vi "PH_gentec_P-Link.Action get and set current Settings for the first Time.vi"(0 "i ref in":refnum<vi>, 5 "error in":errorcluster) -> (14 "i ref out":refnum<vi>, 19 "error out":errorcluster)   [LabVIEW 2014, in "PH_gentec_P-Link.lvlib"]
doc: "This VI gets and sets all current settings for the first time."
uses:
  PH_gentec_P-Link.lvlib
  PH_Basics/PH_Powermeter_BaseClass/PH_Powermeter_BaseClass.State.ctl
  PH_Basics/PH_Powermeter_BaseClass/PH_gentec_BaseClass.Head Settings.ctl
  PH_Basics/PH_Powermeter_BaseClass/PH_Powermeter_BaseClass.lvlib
  instr.lib/Gentec-P-Link/gentec-P-Link - Driver.lvlib
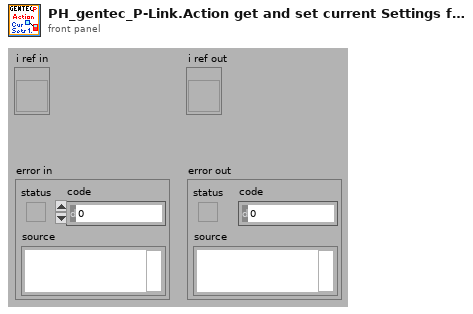
[diagram p1: front panel]
types:
  T1 = typedef "PH_Powermeter_BaseClass.lvlib/PH_gentec_BaseClass.Head Settings.ctl" = cluster{"Trigger Level":dbl, "Wavelength":u32, "Range":u32}
  T2 = typedef "PH_Powermeter_BaseClass.lvlib/PH_Powermeter_BaseClass.State.ctl" = enum32{"off", "operating", "opened", "checked", "connected", "Sets to change", "running"}
  T3 = typedef "PH_Powermeter_BaseClass.lvlib/PH_Powermeter_BaseClass.i attribute.ctl" = cluster{"GUI References":T4, "Connection":T5, "Head Attributes":T6, "VISA resource":refnum<visa-resource-name>, "Energy":T7, "Service ID Energy":i32, "Wanted Settings":T1, "Current Settings":T1}
  T4 = typedef "PH_Powermeter_BaseClass.lvlib/PH_Powermeter_BaseClass.GUI Refs.ctl" = cluster{"Head Attributes":refnum<vi>, "Energy":refnum<vi>, "Connection":refnum<vi>, "VISA Resource":refnum<vi>, "Scaling Factor":refnum<vi>, "Range":refnum<vi>, "Wavelength":refnum<vi>, "Trigger Level":refnum<vi>, "Wanted Settings":refnum<vi>, "Current Settings":refnum<vi>}
  T5 = typedef "PH_Powermeter_BaseClass.lvlib/PH_Powermeter_BaseClass.Connection.ctl" = cluster{"failed checks":i8, "Timeout":bool, "Data read":string, "Failure":bool, "Error":bool, "State":T2}
  T6 = typedef "PH_Powermeter_BaseClass.lvlib/PH_Powermeter_BaseClass.Head Attributes.ctl" = cluster{"Instrument Type":string, "Head Version":string, "Head Name":string, "Serial Number":string, "Firmware":string, "Sensor Type":string, "MinimumRange":u32, "Maximum Range":u32, "Min Wavelength":i32, "Max Wavelength":i32}
  T7 = typedef "PH_Powermeter_BaseClass.lvlib/PH_Powermeter_BaseClass.Energy.ctl" = cluster{"current Value":dbl, "unscaled":dbl, "Scaling Factor":dbl}
  T8 = typedef "PH_gentec_P-Link.lvlib/PH_gentec_P-Link.i attribute.ctl" = cluster{"GUI References":cluster{"Wanted Head Settings":refnum<vi>, "Current Head Settings":refnum<vi>, "Set Auto Range":refnum<vi>, "Trigger Polarity":refnum<vi>, "Trigger Source":refnum<vi>, "Waveform Averages":refnum<vi>, "Continuous":refnum<vi>, "get one Value":refnum<vi>, "Set Zero":refnum<vi>}, "Wanted Head Settings":T9, "Current Head Settings":T9}
  T9 = typedef "PH_gentec_P-Link.lvlib/PH_gentec_P-Link.Head Settings.ctl" = cluster{"Enable Anticipation":bool, "Set Auto Range":bool, "Set Zero":i32, "Current":i32, "Start Data Flow":bool}
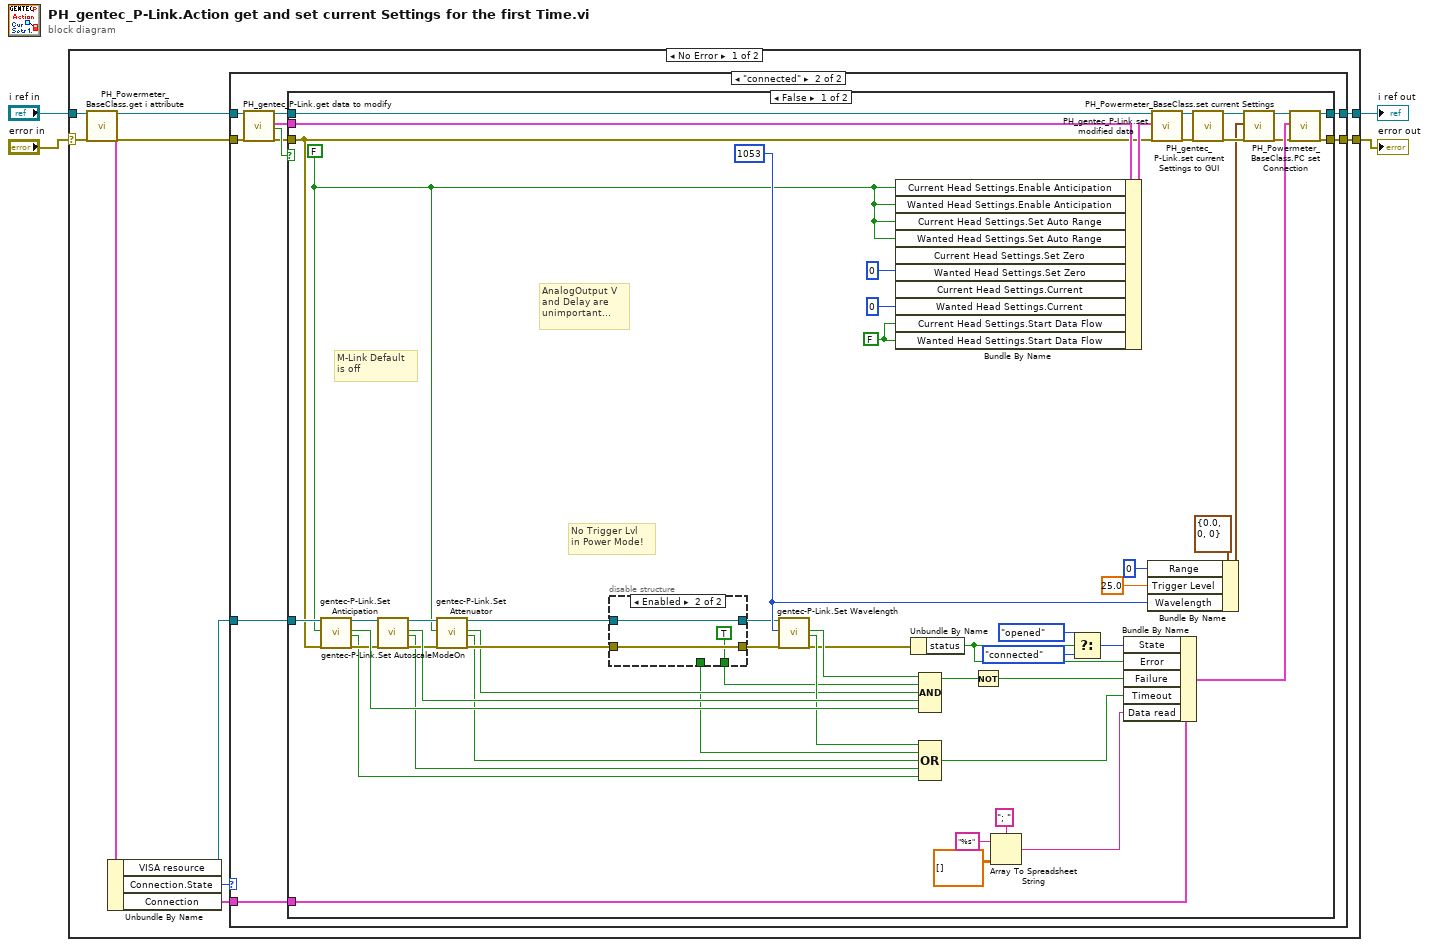
[diagram p0: block diagram]
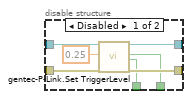
[diagram p3: hidden frame]
diagram:
  n1 = case shown="No Error" "error in" {
    selector: "error in" -> [w5 w93]
    tunnel: [w14 w93] -> w4
    tunnel: [w13 w94] -> w3
    tunnel: "i ref in" -> [w12 w94]
    frame No Error {
      n2 = call "PH_Powermeter_BaseClass.get i attribute.vi"("i ref in"=w12, "error in (no error)"=w5) -> ("i ref out"=w8:refnum<vi>, "i attribute"=w11:T3, "error out"=w7:errorcluster)  [unwired: 15 in]
      n3 = Unbundle By Name(w11) -> ("VISA resource"=w6:refnum<visa-resource-name>, "Connection.State"=w10:T2, "Connection"=w9:T5)
      n4 = case shown="\"connected\"" w10 {
        tunnel: [w15 w17] -> w14
        tunnel: [w16 w18] -> w13
        tunnel: w6 -> [_ w22]
        tunnel: w8 -> [w16 w21]
        tunnel: w7 -> [w15 w20]
        tunnel: w9 -> [_ w19]
        frame Default {
        }
        frame "connected" {
          n5 = call "PH_gentec_P-Link.get data to modify.vi"("i ref in"=w21, "error in (no error)"=w20) -> ("i ref out"=w24:refnum<vi>, "i attribute"=w25:T8, "timed out"=w26:bool, "error out"=w23:errorcluster)  [unwired: 14 in]
          n6 = case shown="False" w26 {
            tunnel: w22 -> [w61 _]
            tunnel: [w66 w92] -> w18
            tunnel: [w65 w91] -> w17
            tunnel: w23 -> [w60 w91]
            tunnel: w24 -> [w80 w92]
            tunnel: w25 -> [w77 _]
            tunnel: w19 -> [w71 _]
            frame False {
              w28 = 0 ("Current Head Settings.Current Measurement")
              w29 = FALSE ("Current Head Settings.Start Data Flow")
              w40 = u16 1053 ("Lambda")
              w27 = 0 ("Current Head Settings.Set Zero")
              w30 = FALSE ("Enable Anticipation")
              # "No Trigger Lvl\nin Power Mode!"
              # "AnalogOutput V\nand Delay are\nunimportant..."
              # "M-Link Default\nis off"
              n7 = call "gentec-P-Link.Set Anticipation.vi"("VISA resource name"=w61, "On/Off"=w30, "error in (no error)"=w60) -> ("VISA resource name"=w58:refnum<visa-resource-name>, "Sucess?"=w59:bool, "TimeOut?"=w53:bool, "error out"=w57:errorcluster)  [unwired: 13 in]
              n8 = call "gentec-P-Link.Set AutoscaleModeOn.vi"("VISA resource name"=w58, "error in (no error)"=w57) -> ("VISA resource name"=w55:refnum<visa-resource-name>, "Sucess?"=w56:bool, "TimeOut?"=w52:bool, "error out"=w54:errorcluster)  [unwired: 14 in]
              n9 = call "gentec-P-Link.Set Attenuator.vi"("VISA resource name"=w55, "On/Off"=w30, "error in (no error)"=w54) -> ("VISA resource name"=w37:refnum<visa-resource-name>, "Sucess?"=w34:bool, "TimeOut?"=w32:bool, "error out"=w39:errorcluster)  [unwired: 13 in]
              n10 = disable-structure shown="Enabled" {
                disable-tunnel: w39 -> [w87 w89]
                disable-tunnel: [w86 w89] -> w38
                disable-tunnel: w37 -> [w85 w90]
                disable-tunnel: [w84 w90] -> w36
                disable-tunnel: [w83 TRUE ("Sucess?")] -> w33
                disable-tunnel: [w82 _] -> w31
                frame Disabled {
                  n11 = call "gentec-P-Link.Set TriggerLevel.vi"("VISA resource name"=w85, "TriggerLevel (J)"=0.25, "error in (no error)"=w87) -> ("VISA resource name"=w84:refnum<visa-resource-name>, "Sucess?"=w83:bool, "TimeOut?"=w82:bool, "error out"=w86:errorcluster)  [unwired: 13 in]
                }
                frame Enabled {
                }
              }
              n12 = call "gentec-P-Link.Set Wavelength.vi"("VISA resource name"=w36, "Wavelength (nm)"=w40, "error in (no error)"=w38) -> ("Sucess?"=w51:bool, "TimeOut?"=w50:bool, "error out"=w49:errorcluster)  [unwired: 13 in, 1 out]
              n13 = Bundle By Name(cluster=w77, "Current Head Settings.Enable Anticipation"=w30, "Wanted Head Settings.Enable Anticipation"=w30, "Current Head Settings.Set Auto Range"=w30, "Wanted Head Settings.Set Auto Range"=w30, "Current Head Settings.Set Zero"=w27, "Wanted Head Settings.Set Zero"=w27, "Current Head Settings.Current"=w28, "Wanted Head Settings.Current"=w28, "Current Head Settings.Start Data Flow"=w29, "Wanted Head Settings.Start Data Flow"=w29) -> (w76:T8)
              n14 = Unbundle By Name(w49) -> ("status"=w69:bool)
              n15 = Compound Arithmetic op=AND(w51, w33, w34, w56, w59) -> (w75:bool)
              n16 = Compound Arithmetic op=OR(w50, w31, w32, w52, w53) -> (w73:bool)
              n17 = Not(x=w75) -> (.not. x?=w72:bool)
              n18 = Array To Spreadsheet String(delimiter (Tab)="; ", array=dbl[][] [], 3:"%s" ("format string")) -> (spreadsheet string=w74:string)
              n19 = Select(t=PH_Powermeter_BaseClass.State."opened" ("State"), s=w69, f=PH_Powermeter_BaseClass.State."connected") -> (s? t:f=w67:T2)
              n20 = Bundle By Name(cluster=w71, "State"=w67, "Error"=w69, "Failure"=w72, "Timeout"=w73, "Data read"=w74) -> (w64:T5)
              n21 = Bundle By Name(cluster=T1 {"Trigger Level"=0.0, "Wavelength"=0, "Range"=0} ("Current Settings"), "Range"=u32 0, "Trigger Level"=25.0, "Wavelength"=w40) -> (w42:T1)
              n22 = call "PH_gentec_P-Link.set modified data.vi"("i ref in"=w80, "i attribute"=w76, "error in (no error)"=w60) -> ("i ref out"=w63:refnum<vi>, "error out"=w62:errorcluster)  [unwired: 15 in]
              n23 = call "PH_gentec_P-Link.set current Settings to GUI.vi"("i ref in"=w63, "error in"=w62) -> ("i ref out"=w45:refnum<vi>, "error out"=w46:errorcluster)  [unwired: 16 in]
              n24 = call "PH_Powermeter_BaseClass.set current Settings.vi"("VI in"=w45, "Current Settings"=w42, "error in (no error)"=w46) -> ("VI out"=w44:refnum<vi>, "error out"=w43:errorcluster)  [unwired: 15 in]
              n25 = call "PH_Powermeter_BaseClass.PC set Connection.vi"("VI in"=w44, "Connection"=w64, "error in (no error)"=w43) -> ("VI out"=w66:refnum<vi>, "error out"=w65:errorcluster)  [unwired: 15 in]
            }
            frame True {
            }
          }
        }
      }
    }
    frame Error {
    }
  }
  "error out" <- w4
  "i ref out" <- w3
